vi "GVMetavariablen.vi"() -> ()   [LabVIEW 2017]
panel:
  in  "MV-Festhalten":bool[](array[boolean])
  in  "MV-Vorgaben":dbl[](array[numeric])
  out "Metavariablen":dbl[](array[numeric])
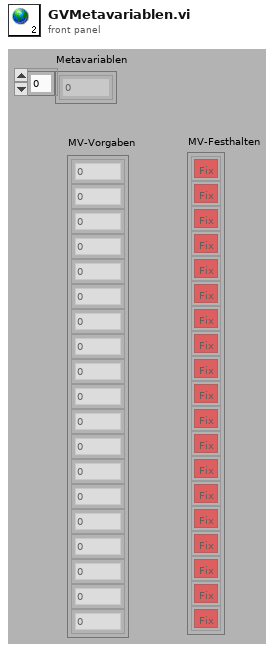
[diagram p1: front panel]
diagram:
